vi "FlatandStackedSequences.vi"() -> ()   [LabVIEW 2020]
panel:
  in  "x 4":dbl=1.0
  out "x+y 2":dbl
  in  "x 3":dbl=1.0
  out "x+y":dbl
  in  "x 2":dbl=1.0
  in  "x":dbl=1.0
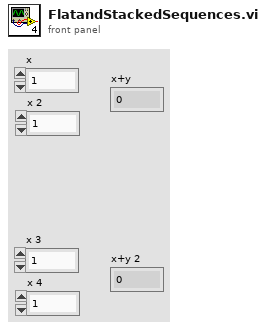
[diagram p1: front panel]
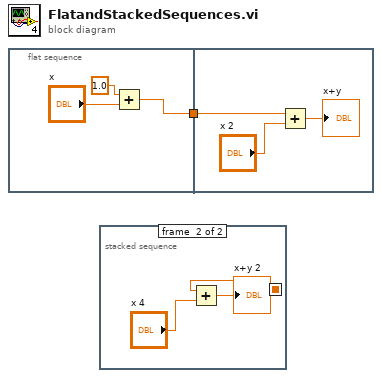
[diagram p0: block diagram]
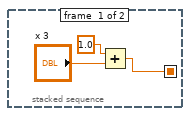
[diagram p2: hidden frame]
diagram:
  n1 = flat-sequence {
    tunnel: [w2] -> w1
    tunnel: w1 -> [w5]
    frame #0 {
      n2 = Add(x=1.0, y="x") -> (x+y=w2:dbl)
    }
    frame #1 {
      n3 = Add(x=w5, y="x 2") -> (x+y=→"x+y":dbl)
    }
  }
  n4 = stacked-sequence {
    seq-local: [w8 _] -> [_ w11]
    frame #0 {
      n5 = Add(x=1.0, y="x 3") -> (x+y=w8:dbl)
    }
    frame #1 {
      n6 = Add(x=w11, y="x 4") -> (x+y=→"x+y 2":dbl)
    }
  }
